vi "ProcessName.vi"() -> (1 "process name":string)   [LabVIEW 2017, in "SinglePointClock.lvlib"]
uses:
  <vilib>/addons/InsightCM/Devices/Shared/Common/SinglePointClock/SinglePointClock.lvlib
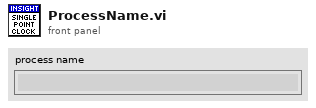
[diagram p1: front panel]
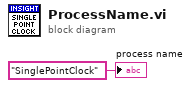
[diagram p0: block diagram]
diagram:
  "process name" <- "SinglePointClock" ("ProcessName")
